vi "Configure Trigger (Edge).vi"(0 "VISA resource name":refnum<visa-resource-name>, 2 "Trigger Level (0)":dbl, 5 "Source (1: Channel 1)":i32(ring)=1 items=["Channel 1"=1, "Channel 2"=2, "Channel 3"=3, "Channel 4"=4, "External"=5, "AC Line"=6], 9 "Edge Type (0: Positive)":i32(ring) items=["Positive", "Negative", "Either"], 11 "error in (no error)":errorcluster) -> (4 "VISA resource name out":refnum<visa-resource-name>, 15 "error out":errorcluster)   [LabVIEW 2015, in "ZhiYuan ZDS Series for TCP.lvlib"]
doc: "Configures the edge setting for trigger."
uses:
  ZhiYuan ZDS Series for TCP.lvlib
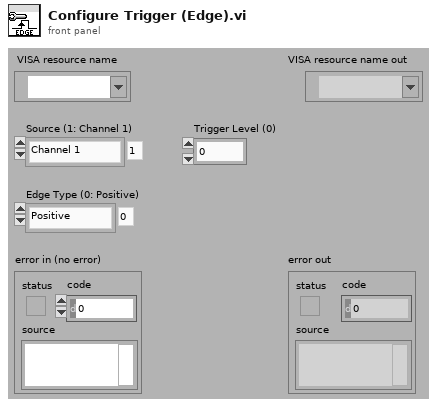
[diagram p1: front panel]
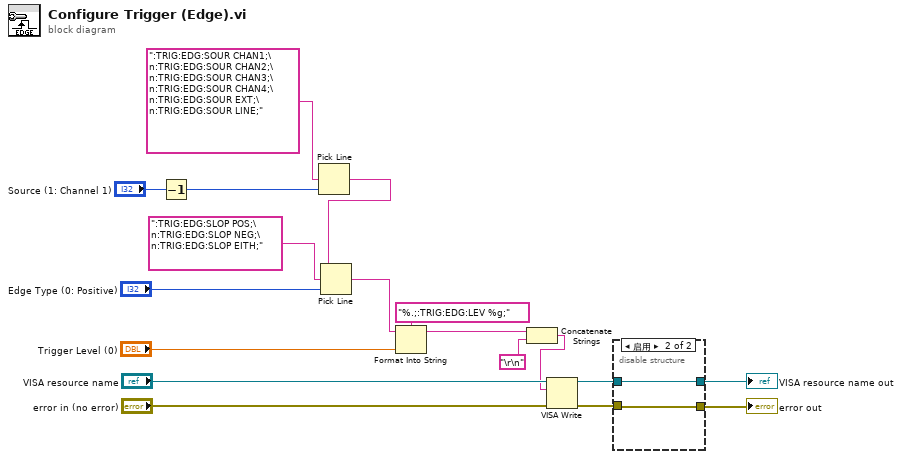
[diagram p0: block diagram]
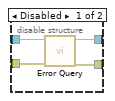
[diagram p2: hidden frame]
diagram:
  n1 = Decrement(x="Source (1: Channel 1)") -> (x-1=w3:i32)
  n2 = Pick Line(multi-line string=":TRIG:EDG:SOUR CHAN1;\n:TRIG:EDG:SOUR CHAN2;\n:TRIG:EDG:SOUR CHAN3;\n:TRIG:EDG:SOUR CHAN4;\n:TRIG:EDG:SOUR EXT;\n:TRIG:EDG:SOUR LINE;", line index=w3) -> (output string=w2:string)  [unwired: 1 in]
  n3 = Pick Line(string ("")=w2, multi-line string=":TRIG:EDG:SLOP POS;\n:TRIG:EDG:SLOP NEG;\n:TRIG:EDG:SLOP EITH;", line index="Edge Type (0: Positive)") -> (output string=w16:string)
  n4 = Format Into String(format string="%.;:TRIG:EDG:LEV %g;", initial string=w16, "Trigger Level (0)") -> (resulting string=w1:string)  [unwired: 1 in, 1 out]
  n5 = Concatenate Strings(w1, "\r\n") -> (w5:string)
  n6 = VISA Write(VISA resource name="VISA resource name", write buffer=w5, error in (no error)="error in (no error)") -> (VISA resource name out=w10:refnum<visa-resource-name>, error out=w9:errorcluster)  [unwired: 1 out]
  n7 = disable-structure shown="启用" {
    disable-tunnel: w10 -> [w22 w24]
    disable-tunnel: w9 -> [w21 w23]
    disable-tunnel: [w20 w24] -> w8
    disable-tunnel: [w19 w23] -> w7
    frame Disabled {
      n8 = call "Error Query.vi"("error in (no error)"=w21, "VISA resource name"=w22) -> ("error out"=w19:errorcluster, "VISA resource name out"=w20:refnum<visa-resource-name>)  [unwired: 6 in, 2 out]
    }
    frame Enabled {
    }
  }
  "VISA resource name out" <- w8
  "error out" <- w7
